vi "Is String.vi"(11 "Input String":string) -> (3 "Is String?":bool)   [LabVIEW 2019, in "SLL JSON to Cluster.lvlib"]
doc: "This VI returns true if the input is string,\n\"123\" => True\n123 => False"
uses:
  SLL JSON to Cluster.lvlib
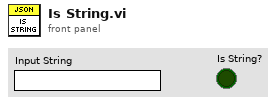
[diagram p1: front panel]
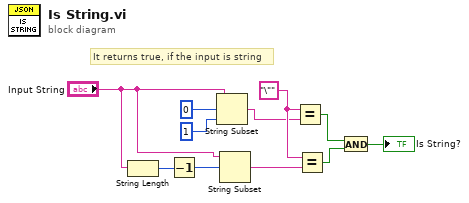
[diagram p0: block diagram]
diagram:
  w11 = "\"" ("x")
  # "It returns true, if the input is string"
  n1 = String Length(string="Input String") -> (length=w7:i32)
  n2 = Decrement(x=w7) -> (x-1=w9:i32)
  n3 = String Subset(string="Input String", offset (0)=0, length (rest)=1 ("length (rest)")) -> (substring=w8:string)
  n4 = String Subset(string="Input String", offset (0)=w9) -> (substring=w10:string)  [unwired: 1 in]
  n5 = Equal?(x=w11, y=w8) -> (x = y?=w4:bool)
  n6 = Equal?(x=w11, y=w10) -> (x = y?=w3:bool)
  n7 = And(x=w4, y=w3) -> (x .and. y?=→"Is String?":bool)
